vi "Keyence.Cmd.Reset.vi"(8 "error in (no error)":errorcluster, 9 "Timeout [ms] (1000)":i32=1000, 11 "connection ID":refnum<k5>) -> (0 "error out":errorcluster, 3 "connection ID out":refnum<k5>)   [LabVIEW 2016]
panel:
  out "response":string
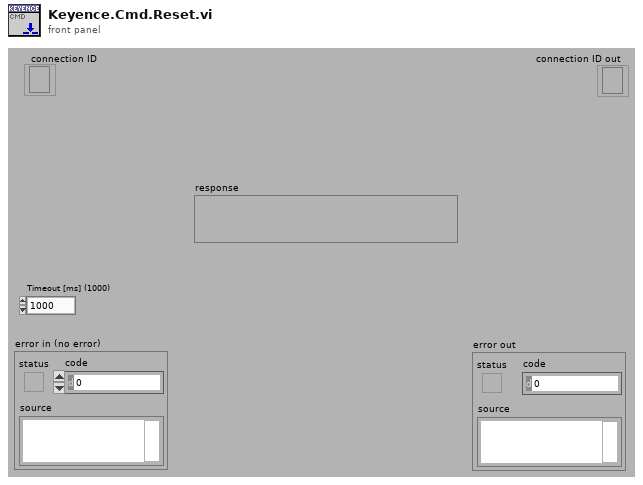
[diagram p1: front panel]
types:
  T1 = enum16{"Standard", "Buffered", "CRLF", "Immediate"}
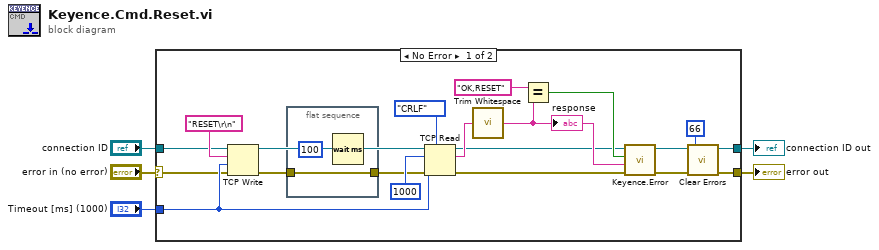
[diagram p0: block diagram]
diagram:
  n1 = case shown="No Error" "error in (no error)" {
    selector: "error in (no error)" -> [w9 w27]
    tunnel: [w7 w27] -> w5
    tunnel: "Timeout [ms] (1000)" -> [w12 _]
    tunnel: "connection ID" -> [w10 w26]
    tunnel: [w8 w26] -> w1
    frame No Error {
      n2 = TCP Write(connection ID=w10, data in="RESET\r\n" ("concatenated string"), error in (no error)=w9, 9:w12) -> (connection ID out=w23:refnum<k5>, error out=w20:errorcluster)  [unwired: 1 out]
      n3 = flat-sequence {
        tunnel: w20 -> [w25]
        tunnel: [w25] -> w19
        frame #0 {
          n4 = Wait (ms)(milliseconds to wait=u32 100) -> ()  [unwired: 1 out]
        }
      }
      n5 = TCP Read(connection ID=w23, bytes to read=1000, error in (no error)=w19, 7:T1."CRLF" ("mode (standard)"), 9:w12) -> (connection ID out=w8:refnum<k5>, data out=w16:string, error out=w15:errorcluster)
      n6 = call <vilib>:"Trim Whitespace.vi"("string"=w16) -> ("trimmed string"=w11:string)  [unwired: 1 in]
      "response" <- w11
      n7 = Equal?(x="OK,RESET", y=w11) -> (x = y?=w13:bool)
      n8 = call "Keyence.Error.vi"("error in (no error)"=w15, "Response"=w11, "Cmd ok"=w13) -> ("error out"=w14:errorcluster)  [unwired: 8 in]
      n9 = call <vilib>:"Clear Errors.vi"("error in (no error)"=w14, "specific error code to clear (0: all)"=66) -> ("error out"=w7:errorcluster)  [unwired: 4 in, 1 out]
    }
    frame Error {
    }
  }
  "error out" <- w5
  "connection ID out" <- w1
